vi "Read.vi"(11 "Plot Group Events Value in":refnum<class "Plot Group Events Value.lvclass">) -> (2 "Plot Group":refnum<event-registration>)   [LabVIEW 2020, in "VolatusGUI.lvlib" / "Plot Group Events Value.lvclass"]
uses:
  Plot Group Events Value.lvclass
  Plot Group Events Value.lvclass/Plot Group Events Value.ctl
  Historian Charting Manager/X-Axis Type.ctl
  Historian Charting Manager/Historian Charting Manager.lvclass
  Historian Charting Manager/Scale.ctl
  Historian Charting Manager/Plot Config.ctl
  Historian Charting Manager/Plot Group Config.ctl
  Historian Charting Manager/Plot Group Changed Data.ctl
  Historian Charting Manager/Plot Group Removed Data.ctl
  Historian Charting Manager/New Plot Group Data.ctl
  Historian Charting Manager/Plot Group Events.ctl
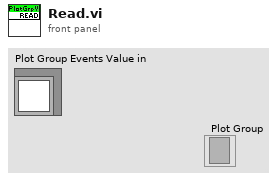
[diagram p1: front panel]
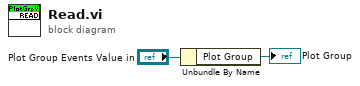
[diagram p0: block diagram]
diagram:
  n1 = Unbundle By Name("Plot Group Events Value in") -> ("Plot Group"=→"Plot Group":refnum<event-registration>)
